vi "Get Stats.vi"(8 "error in (no error)":errorcluster, 11 "Team Dashboard Panel in":refnum<class "Team Dashboard Panel.lvclass">) -> (0 "error out":errorcluster, 2 "Team Stats":T1, 3 "Team Dashboard Panel out":refnum<class "Team Dashboard Panel.lvclass">)   [LabVIEW 2020, in "SB App.lvlib" / "Team Dashboard Panel.lvclass"]
uses:
  Team Dashboard Panel.lvclass
  SquareBattle/Team Stats.ctl
  Team Dashboard Panel.lvclass/Team Dashboard Panel.ctl
  SquareBattle/SquareBattle.lvlib
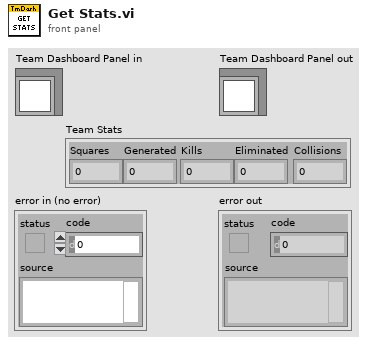
[diagram p1: front panel]
types:
  T1 = typedef "SquareBattle.lvlib/Team Stats.ctl" = cluster{"Squares":i32, "Generated":i32, "Kills":i32, "Eliminated":i32, "Collisions":i32}
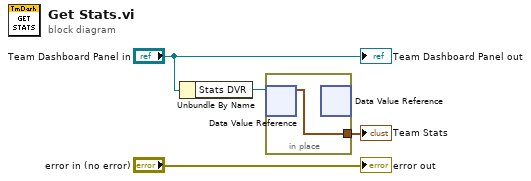
[diagram p0: block diagram]
diagram:
  n1 = Unbundle By Name("Team Dashboard Panel in") -> ("Stats DVR"=w3:refnum<data-value>)
  n2 = in-place {
    in-place-border: [w5] -> w1
    n3 = in-place-dvr #1(w3) -> (w5:T1)  [unwired: 1 out]
    n4 = in-place-dvr #1() -> ()  [unwired: 1 in, 2 out]
  }
  "Team Stats" <- w1
  "error out" <- "error in (no error)"
  "Team Dashboard Panel out" <- "Team Dashboard Panel in"
